vi "UsrProfiles-Check profile exists.vi"(8 "error in":errorcluster, 11 "Profile file path":path) -> (0 "error out":errorcluster, 1 "Profile's file path":path, 3 "Profile file exists":bool)   [LabVIEW 2017]
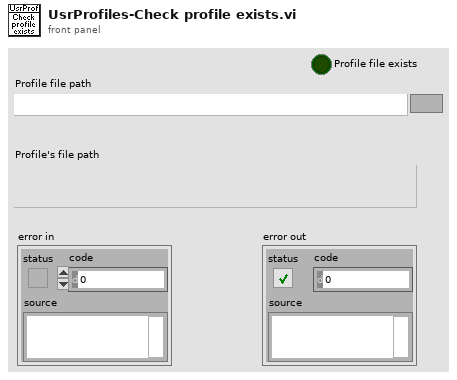
[diagram p1: front panel]
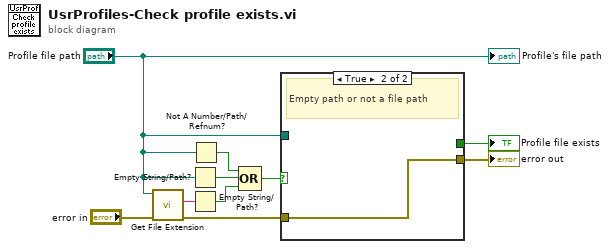
[diagram p0: block diagram]
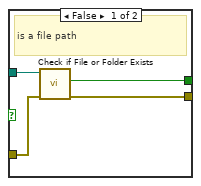
[diagram p2: hidden frame]
diagram:
  n1 = call <vilib>:"Get File Extension.vi"("error in (no error)"="error in", "file"="Profile file path") -> ("error out"=w8:errorcluster, "lowercase file extension"=w4:string)  [unwired: 5 in, 3 out]
  n2 = Empty String/Path?(string/path="Profile file path") -> (empty?=w5:bool)
  n3 = Empty String/Path?(string/path=w4) -> (empty?=w6:bool)
  n4 = Not A Number/Path/Refnum?(number/path/refnum="Profile file path") -> (NaN/Path/Refnum?=w9:bool)
  n5 = Compound Arithmetic op=OR(w9, w5, w6) -> (w7:bool)
  n6 = case shown="True" w7 {
    tunnel: "Profile file path" -> [w14 _]
    tunnel: w8 -> [w13 w15]
    tunnel: [w12 _] -> w10
    tunnel: [w11 w15] -> w3
    frame False {
      # "is a file path"
      n7 = call <vilib>:"Check if File or Folder Exists.vi"("error in (no error)"=w13, "path"=w14) -> ("error out"=w11:errorcluster, "file or folder exists?"=w12:bool)  [unwired: 7 in, 1 out]
    }
    frame True {
      # "Empty path or not a file path"
    }
  }
  "Profile file exists" <- w10
  "error out" <- w3
  "Profile's file path" <- "Profile file path"
